vi "ref_Chirp cmd_DOB coeffs2.vi"() -> ()   [LabVIEW 2014]
uses:
  <vilib>/rvi/Analysis/host/Butterworth/config/Butterworth Filter Order.ctl
  <vilib>/rvi/Analysis/host/Butterworth/config/Butterworth Filter Type.ctl
  <vilib>/FPGAPlugInAG/cRIO-9039/niLvFpga_Open_cRIO-9039.vi
  <vilib>/rvi/interface/common/dynamic/niFpgaDynamicAddResources.vi
  <vilib>/rvi/Analysis/host/Butterworth/config/BwScaledCoefficients.vi
  <vilib>/Utility/error.llb/Error Cluster From Error Code.vi
  <vilib>/rvi/errors/niLvFpgaAdjustHostInterfaceError.vi
  <vilib>/FPGAPlugInAG/Dynamic/niLvFpga_Close_Dynamic.vi
  <vilib>/rvi/interface/nirviOpenFPGA/nirviOpenFPGA.xnode
  FPGA Bitfiles/forcecontroledu_FPGATarget_impedancecontrol_ddnKbnGE22E.lvbitx
  FPGA VIs/impedance_control_DOB_one motor_final_2.vi
  <vilib>/rvi/Analysis/host/Butterworth/XNode/ButterworthCoefficients.xnode
  <vilib>/rvi/interface/nirviReadWriteControl/nirviReadWriteControl.xnode
  <vilib>/rvi/interface/nirviCloseFPGA/nirviCloseFPGA.xnode
  <vilib>/rvi/interface/Simulation/niFpgaSimulationCallBeginRW.vi
  <vilib>/rvi/Analysis/host/Public/NI_FpgaMspHost.lvlib
  NiFpgaLv.dll
panel:
  in  "DOB gain1 (20)":bool
  out "Pn_inv*Q output":sgl
  in  "b0":sgl
  in  "b1":sgl
  in  "b2":sgl
  in  "b3":sgl
  in  "a1":sgl
  in  "a0":sgl
  in  "a2":sgl
  in  "a3":sgl
  out "f (N)":fxp<+/-,30,11>
  in  "Step form 1":bool
  in  "Step offset":sgl format="%#_25g"
  in  "Step size":sgl
  out "fd step cmd":sgl format="%#_6f"
  in  "Step form 2":bool
  in  "Coeffs ini":bool
  in  "wq (rad/s)":dbl=0.795775
  in  "DOB Stop":bool
  out "Target time finished":bool
  in  "Target time (s)":sgl min=0 max=10800
  in  "Initial freq (Hz)":sgl min=0 max=200
  in  "Target freq (Hz)":sgl min=0 max=200
  in  "Chirp type (exp/linear)":bool
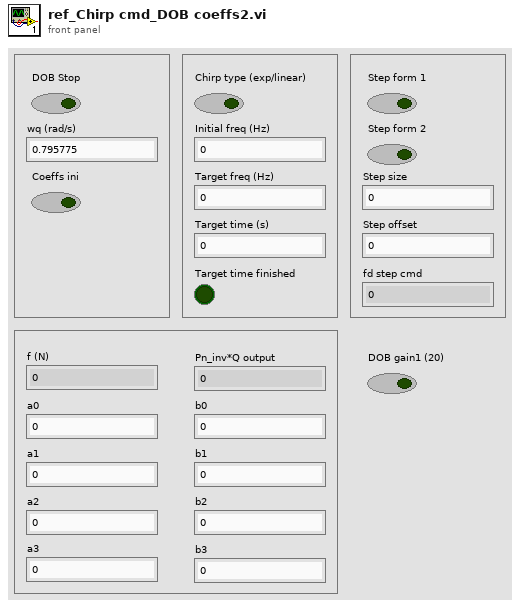
[diagram p1: front panel]
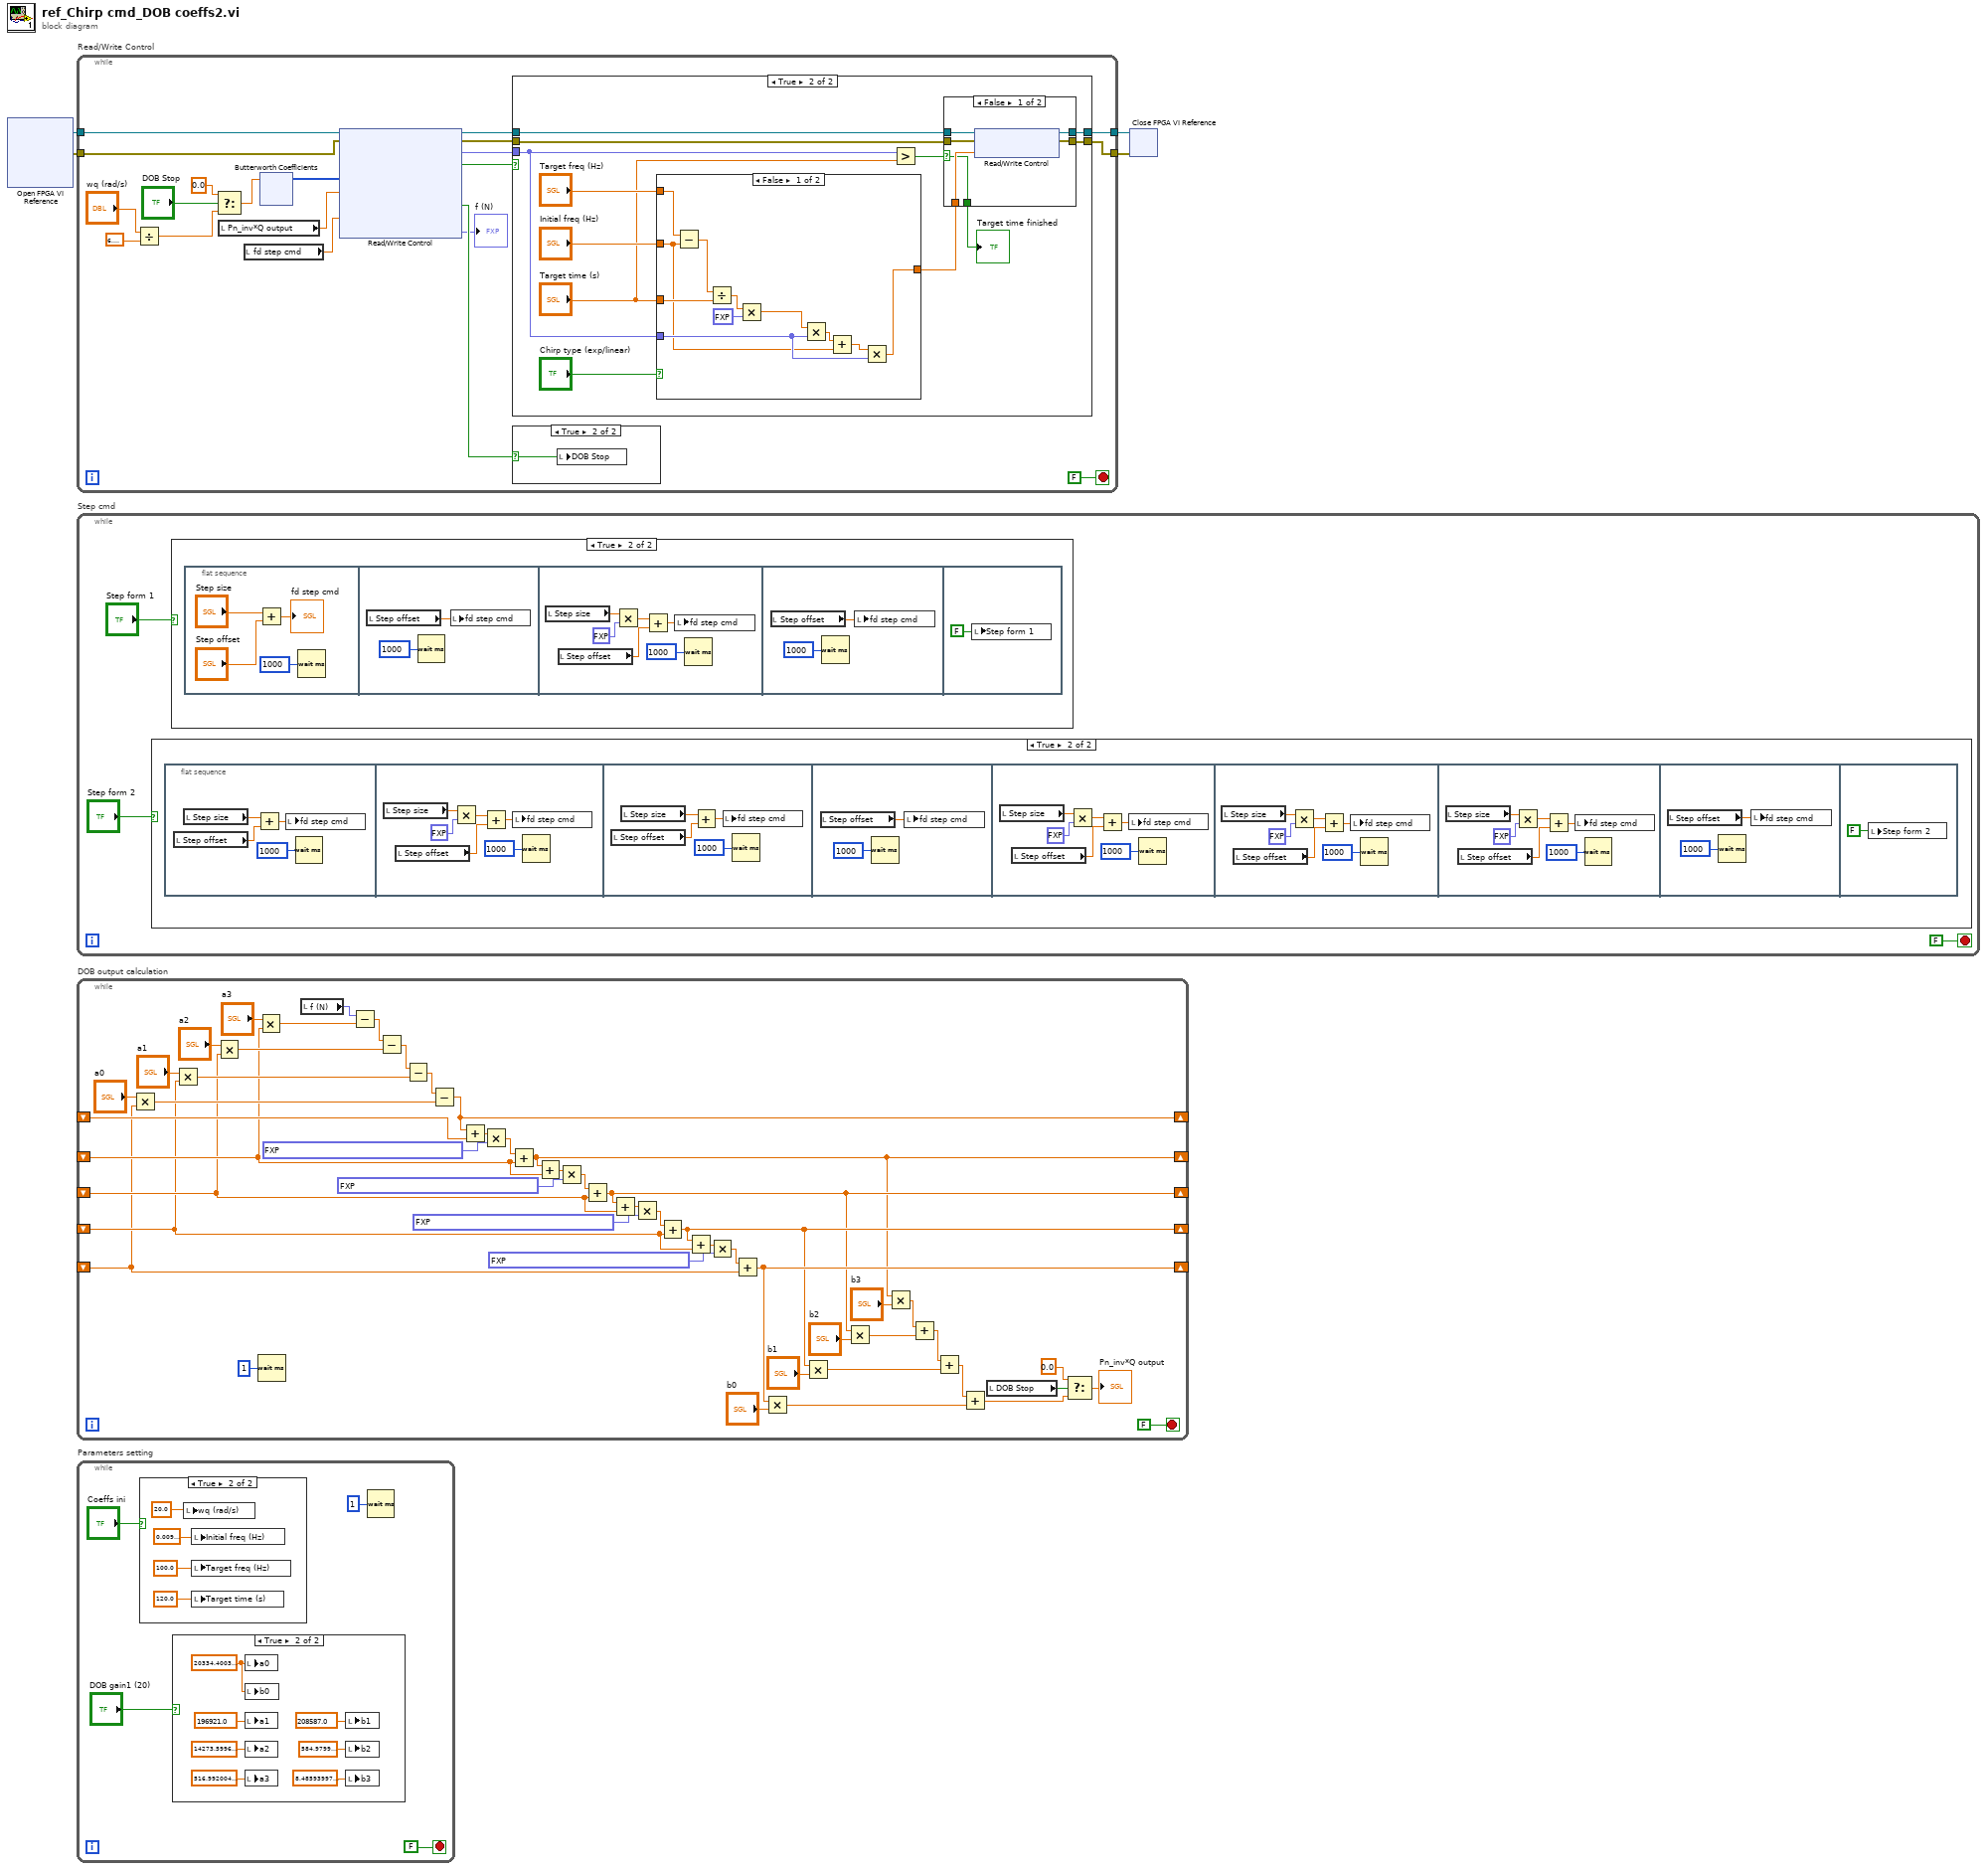
[diagram p0: block diagram]
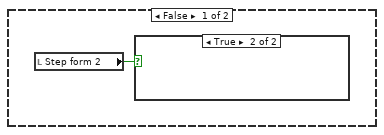
[diagram p2: hidden frame]
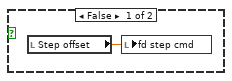
[diagram p3: hidden frame]
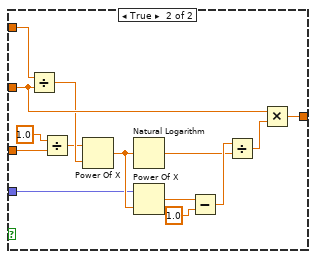
[diagram p10: hidden frame]
diagram:
  n1 = xnode "Open FPGA VI Reference"() -> ("FPGA VI Reference Out"=w2:refnum<k20>, "error out"=w1:errorcluster)  [unwired: 2 in]
  n2 = while "Read/Write Control" {
    tunnel: [w22] -> w4
    tunnel: [w21] -> w3
    tunnel: w2 -> [w24]
    tunnel: w1 -> [w23]
    stop <- FALSE stop-if-true
    n3 = Divide(x="wq (rad/s)", y=6.283185307179586) -> (x/y=w13:dbl)
    n4 = Select(t=0.0, s="DOB Stop", f=w13) -> (s? t:f=w14:dbl)
    n5 = local read "Pn_inv*Q output"() -> (w5:sgl)
    n6 = local read "fd step cmd"() -> (w7:sgl)
    n7 = xnode "Butterworth Coefficients"("cutoff frequency (Hz)"=w14) -> ("scaled coefficients"=w10:i32[])  [unwired: 2 in, 1 out]
    n8 = xnode "Read/Write Control"("FPGA VI Reference In"=w24, "error in"=w23, "Q filter coe"=w10, "Pn_inv*Q output"=w5, "fd step size (N)"=w7) -> ("FPGA VI Reference Out"=w20:refnum<k20>, "error out"=w19:errorcluster, "Sine time (s)"=w18:fxp<+,47,13>, "Chirp cmd/const freq"=w17:bool, "Stop Motor"=w9:bool, "f (N)"=→"f (N)":fxp<+/-,30,11>)
    n9 = case shown="True" w17 {
      tunnel: w18 -> [_ w43]
      tunnel: [w34 w39] -> w22
      tunnel: [w33 w38] -> w21
      tunnel: w20 -> [w34 w37]
      tunnel: w19 -> [w33 w36]
      frame False {
      }
      frame True {
        n10 = case shown="False" "Chirp type (exp/linear)" {
          tunnel: "Target freq (Hz)" -> [w66 w80]
          tunnel: "Initial freq (Hz)" -> [w57 w74]
          tunnel: "Target time (s)" -> [w62 w78]
          tunnel: [w60 w73] -> w40
          tunnel: w43 -> [w58 w67]
          frame False {
            n11 = Subtract(x=w66, y=w57) -> (x-y=w65:sgl)
            n12 = Divide(x=w65, y=w62) -> (x/y=w56:sgl)
            n13 = Multiply(x=w56, y=fxp<+,1,0> 0.5) -> (x*y=w59:sgl)
            n14 = Multiply(x=w59, y=w58) -> (x*y=w63:sgl)
            n15 = Add(x=w63, y=w57) -> (x+y=w61:sgl)
            n16 = Multiply(x=w61, y=w58) -> (x*y=w60:sgl)
          }
          frame True {
            n17 = Divide(x=w80, y=w74) -> (x/y=w72:sgl)
            n18 = Divide(x=sgl 1.0, y=w78) -> (x/y=w71:sgl)
            n19 = Power Of X(1:w72, 2:w71) -> (0:w69:sgl)
            n20 = Natural Logarithm(1:w69) -> (0:w68:sgl)
            n21 = Power Of X(1:w69, 2:w67) -> (0:w70:sgl)
            n22 = Subtract(x=w70, y=sgl 1.0 ("x")) -> (x-y=w76:sgl)
            n23 = Divide(x=w76, y=w68) -> (x/y=w75:sgl)
            n24 = Multiply(x=w74, y=w75) -> (x*y=w73:sgl)
          }
        }
        n25 = Greater?(x=w43, y="Target time (s)") -> (0:w41:bool)
        n26 = case shown="False" w41 {
          selector: w41 -> [w47 w53]
          tunnel: w40 -> [w48 _]
          tunnel: [w50 w55] -> w39
          tunnel: [w49 w54] -> w38
          tunnel: w37 -> [w52 w55]
          tunnel: w36 -> [w51 w54]
          tunnel: [w47 w53] -> w35
          frame False {
            n27 = xnode "Read/Write Control"("FPGA VI Reference In"=w52, "error in"=w51, "Sine freq (Hz)"=w48) -> ("FPGA VI Reference Out"=w50:refnum<k20>, "error out"=w49:errorcluster)
          }
          frame True {
          }
        }
        "Target time finished" <- w35
      }
    }
    n28 = case shown="True" w9 {
      selector: w9 -> [_ w25]
      frame False {
      }
      frame True {
        n29 = local write "DOB Stop"(w25) -> ()
      }
    }
  }
  n30 = while "Step cmd" {
    stop <- FALSE stop-if-true
    n31 = case shown="True" "Step form 2" {
      frame False {
      }
      frame True {
        n32 = flat-sequence {
          frame #0 {
            n33 = local read "Step offset"() -> (w103:sgl)
            n34 = local read "Step size"() -> (w104:sgl)
            n35 = Add(x=w104, y=w103) -> (x+y=w102:sgl)
            n36 = local write "fd step cmd"(w102) -> ()
            n37 = Wait (ms)(milliseconds to wait=u32 1000) -> ()  [unwired: 1 out]
          }
          frame #1 {
            n38 = local read "Step size"() -> (w110:sgl)
            n39 = local read "Step offset"() -> (w107:sgl)
            n40 = Multiply(x=w110, y=fxp<+,1,2> 2.0) -> (x*y=w108:sgl)
            n41 = Add(x=w108, y=w107) -> (x+y=w106:sgl)
            n42 = local write "fd step cmd"(w106) -> ()
            n43 = Wait (ms)(milliseconds to wait=u32 1000) -> ()  [unwired: 1 out]
          }
          frame #2 {
            n44 = local read "Step offset"() -> (w112:sgl)
            n45 = local read "Step size"() -> (w111:sgl)
            n46 = Add(x=w111, y=w112) -> (x+y=w113:sgl)
            n47 = local write "fd step cmd"(w113) -> ()
            n48 = Wait (ms)(milliseconds to wait=u32 1000) -> ()  [unwired: 1 out]
          }
          frame #3 {
            n49 = local read "Step offset"() -> (w115:sgl)
            n50 = Wait (ms)(milliseconds to wait=u32 1000) -> ()  [unwired: 1 out]
            n51 = local write "fd step cmd"(w115) -> ()
          }
          frame #4 {
            n52 = local read "Step size"() -> (w117:sgl)
            n53 = local read "Step offset"() -> (w120:sgl)
            n54 = Multiply(x=w117, y=fxp<+/-,1,1> -1.0) -> (x*y=w119:sgl)
            n55 = Add(x=w119, y=w120) -> (x+y=w121:sgl)
            n56 = local write "fd step cmd"(w121) -> ()
            n57 = Wait (ms)(milliseconds to wait=u32 1000) -> ()  [unwired: 1 out]
          }
          frame #5 {
            n58 = local read "Step size"() -> (w128:sgl)
            n59 = local read "Step offset"() -> (w125:sgl)
            n60 = Multiply(x=w128, y=fxp<+/-,1,2> -2.0) -> (x*y=w126:sgl)
            n61 = Add(x=w126, y=w125) -> (x+y=w124:sgl)
            n62 = local write "fd step cmd"(w124) -> ()
            n63 = Wait (ms)(milliseconds to wait=u32 1000) -> ()  [unwired: 1 out]
          }
          frame #6 {
            n64 = local read "Step size"() -> (w134:sgl)
            n65 = local read "Step offset"() -> (w131:sgl)
            n66 = Multiply(x=w134, y=fxp<+/-,1,1> -1.0) -> (x*y=w132:sgl)
            n67 = Add(x=w132, y=w131) -> (x+y=w130:sgl)
            n68 = local write "fd step cmd"(w130) -> ()
            n69 = Wait (ms)(milliseconds to wait=u32 1000) -> ()  [unwired: 1 out]
          }
          frame #7 {
            n70 = local read "Step offset"() -> (w136:sgl)
            n71 = Wait (ms)(milliseconds to wait=u32 1000) -> ()  [unwired: 1 out]
            n72 = local write "fd step cmd"(w136) -> ()
          }
          frame #8 {
            n73 = local write "Step form 2"(FALSE ("Step form 2")) -> ()
          }
        }
      }
    }
    n74 = case shown="True" "Step form 1" {
      frame False {
        n75 = local read "Step form 2"() -> (w84:bool)
        n76 = case shown="True" w84 {
          frame False {
            n77 = local read "Step offset"() -> (w85:sgl)
            n78 = local write "fd step cmd"(w85) -> ()
          }
          frame True {
          }
        }
      }
      frame True {
        n79 = flat-sequence {
          frame #0 {
            n80 = Add(x="Step size", y="Step offset") -> (x+y=→"fd step cmd":sgl)
            n81 = Wait (ms)(milliseconds to wait=u32 1000) -> ()  [unwired: 1 out]
          }
          frame #1 {
            n82 = local read "Step offset"() -> (w91:sgl)
            n83 = Wait (ms)(milliseconds to wait=u32 1000) -> ()  [unwired: 1 out]
            n84 = local write "fd step cmd"(w91) -> ()
          }
          frame #2 {
            n85 = local read "Step size"() -> (w97:sgl)
            n86 = local read "Step offset"() -> (w94:sgl)
            n87 = Multiply(x=w97, y=fxp<+/-,1,1> -1.0) -> (x*y=w95:sgl)
            n88 = Add(x=w95, y=w94) -> (x+y=w93:sgl)
            n89 = local write "fd step cmd"(w93) -> ()
            n90 = Wait (ms)(milliseconds to wait=u32 1000) -> ()  [unwired: 1 out]
          }
          frame #3 {
            n91 = local read "Step offset"() -> (w98:sgl)
            n92 = Wait (ms)(milliseconds to wait=u32 1000) -> ()  [unwired: 1 out]
            n93 = local write "fd step cmd"(w98) -> ()
          }
          frame #4 {
            n94 = local write "Step form 1"(FALSE ("Step form 1")) -> ()
          }
        }
      }
    }
  }
  n95 = while "DOB output calculation" {
    shift-right: [w163] -> _
    shift-left: _ -> [w164]
    shift-right: [w144] -> _
    shift-left: _ -> [w162]
    shift-right: [w145] -> _
    shift-left: _ -> [w161]
    shift-right: [w146] -> _
    shift-left: _ -> [w160]
    shift-right: [w147] -> _
    shift-left: _ -> [w159]
    stop <- FALSE stop-if-true
    n96 = Multiply(x="a0", y=w159) -> (x*y=w187:sgl)
    n97 = Multiply(x="a1", y=w160) -> (x*y=w186:sgl)
    n98 = Multiply(x="a2", y=w161) -> (x*y=w183:sgl)
    n99 = Multiply(x="a3", y=w162) -> (x*y=w181:sgl)
    n100 = Wait (ms)(milliseconds to wait=u32 1) -> ()  [unwired: 1 out]
    n101 = local read "f (N)"() -> (w158:fxp<+/-,30,11>)
    n102 = Subtract(x=w158, y=w181) -> (x-y=w173:sgl)
    n103 = Subtract(x=w173, y=w183) -> (x-y=w172:sgl)
    n104 = Subtract(x=w172, y=w186) -> (x-y=w165:sgl)
    n105 = Subtract(x=w165, y=w187) -> (x-y=w163:sgl)
    n106 = Add(x=w163, y=w164) -> (x+y=w166:sgl)
    n107 = Multiply(x=w166, y=fxp<+,20,-10> 0.0005000000819563866) -> (x*y=w168:sgl)
    n108 = Add(x=w168, y=w162) -> (x+y=w144:sgl)
    n109 = Add(x=w144, y=w162) -> (x+y=w169:sgl)
    n110 = Multiply(x=w169, y=fxp<+,20,-10> 0.0005000000819563866) -> (x*y=w171:sgl)
    n111 = Add(x=w171, y=w161) -> (x+y=w145:sgl)
    n112 = Add(x=w145, y=w161) -> (x+y=w176:sgl)
    n113 = Multiply(x=w176, y=fxp<+,20,-10> 0.0005000000819563866) -> (x*y=w174:sgl)
    n114 = Add(x=w174, y=w160) -> (x+y=w146:sgl)
    n115 = Add(x=w146, y=w160) -> (x+y=w177:sgl)
    n116 = Multiply(x=w177, y=fxp<+,20,-10> 0.0005000000819563866) -> (x*y=w179:sgl)
    n117 = Add(x=w179, y=w159) -> (x+y=w147:sgl)
    n118 = Multiply(x=w147, y="b0") -> (x*y=w157:sgl)
    n119 = Multiply(x=w146, y="b1") -> (x*y=w155:sgl)
    n120 = Multiply(x=w145, y="b2") -> (x*y=w153:sgl)
    n121 = Multiply(x=w144, y="b3") -> (x*y=w152:sgl)
    n122 = Add(x=w152, y=w153) -> (x+y=w154:sgl)
    n123 = Add(x=w154, y=w155) -> (x+y=w156:sgl)
    n124 = Add(x=w156, y=w157) -> (x+y=w142:sgl)
    n125 = local read "DOB Stop"() -> (w140:bool)
    n126 = Select(t=sgl 0.0, s=w140, f=w142) -> (s? t:f=→"Pn_inv*Q output":sgl)
  }
  n127 = while "Parameters setting" {
    stop <- FALSE stop-if-true
    n128 = case shown="True" "Coeffs ini" {
      frame False {
      }
      frame True {
        n129 = local write "wq (rad/s)"(20.0 ("wq (rad/s)")) -> ()
        n130 = local write "Initial freq (Hz)"(sgl 0.01 ("Initial freq (Hz)")) -> ()
        n131 = local write "Target freq (Hz)"(sgl 100.0 ("Target freq (Hz)")) -> ()
        n132 = local write "Target time (s)"(sgl 120.0 ("Target time (s)")) -> ()
      }
    }
    n133 = case shown="True" "DOB gain1 (20)" {
      frame False {
      }
      frame True {
        w198 = sgl 20334.4 ("a0")
        n134 = local write "a0"(w198) -> ()
        n135 = local write "b0"(w198) -> ()
        n136 = local write "a1"(sgl 196921.0 ("a1")) -> ()
        n137 = local write "a2"(sgl 14273.6 ("a2")) -> ()
        n138 = local write "a3"(sgl 516.992 ("a3")) -> ()
        n139 = local write "b1"(sgl 208587.0 ("b1")) -> ()
        n140 = local write "b2"(sgl 584.98 ("b2")) -> ()
        n141 = local write "b3"(sgl 8.48594 ("b3")) -> ()
      }
    }
    n142 = Wait (ms)(milliseconds to wait=u32 1) -> ()  [unwired: 1 out]
  }
  n143 = xnode "Close FPGA VI Reference"("FPGA VI Reference In"=w4, "error in"=w3) -> ()  [unwired: 1 out]
